vi "Check for duplicates in csv field.vi"(8 "error in (no error)":errorcluster, 10 "CSV field (0-N)":i32, 11 "multi-line string":string) -> (0 "error out":errorcluster, 1 "lines":i32, 2 "Duplicate Cnt":i32, 3 "Duplicates?":bool, 4 "Sorted array":string[][](array[string]))   [LabVIEW 2013]
panel:
  out "Duplicate data":string[](array[string])
  out "line array":string[][](array[string])
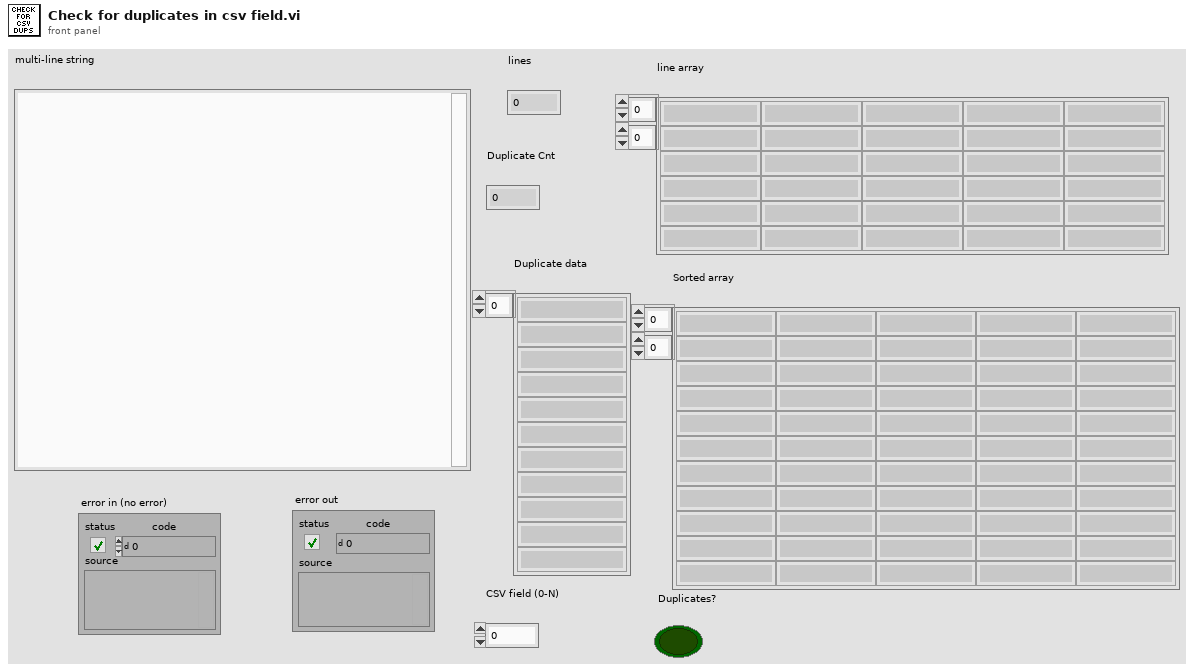
[diagram p1: front panel]
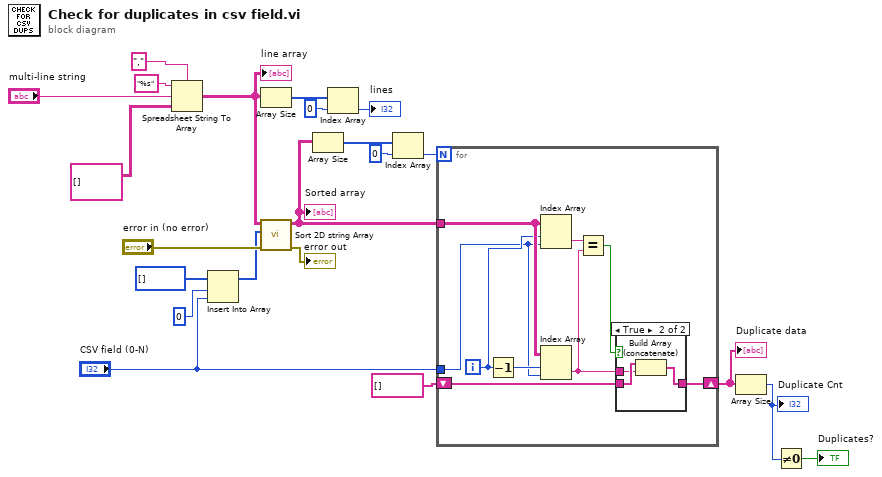
[diagram p0: block diagram]
diagram:
  n1 = Spreadsheet String To Array(delimiter (Tab)=",", format string="%s", spreadsheet string="multi-line string", array type (2D Dbl)=string[][] []) -> (array=w15:string[][])
  "line array" <- w15
  n2 = Insert Into Array(array=i32[] [], index=0, new element="CSV field (0-N)") -> (w1:i32[])
  n3 = Array Size(array=w15) -> (size(s)=w18:i32[])
  n4 = call "Sort 2D string Array.vi"("error in (no error)"="error in (no error)", "Priority Columns (0)"=w1, "Unsorted Array"=w15) -> ("error out"=→"error out":errorcluster, "Sorted array"=w9:string[][])  [unwired: 7 in]
  "Sorted array" <- w9
  n5 = Array Size(array=w9) -> (size(s)=w12:i32[])
  n6 = Index Array(array=w18, index=0) -> (element=→"lines":i32)
  n7 = Index Array(array=w12, index=0) -> (element=w10:i32)
  n8 = for {
    N: w10 -> [_]
    tunnel: w9 -> [w31]
    tunnel: "CSV field (0-N)" -> [w28]
    shift-right: [w24] -> w7
    shift-left: string[] [] -> [w25]
    i -> [w30]
    n9 = Decrement(x=w30) -> (x-1=w29:i32)
    n10 = Index Array(array=w31, index (row)=w30, index (col)=w28) -> (element=w27:string)
    n11 = Index Array(array=w31, index (row)=w29, index (col)=w28) -> (element=w23:string)
    n12 = Equal?(x=w27, y=w23) -> (x = y?=w26:bool)
    n13 = case shown="True" w26 {
      tunnel: w25 -> [w32 w35]
      tunnel: [w32 w33] -> w24
      tunnel: w23 -> [_ w34]
      frame False {
      }
      frame True {
        n14 = Build Array (concatenate)(w35, w34) -> (w33:string[])
      }
    }
  }
  "Duplicate data" <- w7
  n15 = Array Size(array=w7) -> (size(s)=w6:i32)
  "Duplicate Cnt" <- w6
  n16 = Not Equal To 0?(x=w6) -> (x != 0?=→"Duplicates?":bool)
